vi "Reboot Active Target.vi"(8 "error in":errorcluster) -> (0 "error out":errorcluster)   [LabVIEW 2020, in "cRIO System Tests.lvclass"]
uses:
  cRIO System Tests.lvclass
  <vilib>/nisyscfg/nisyscfg.lvlib
  7f296576-305d-4d39-9592-3a047ecdf3ee.vi
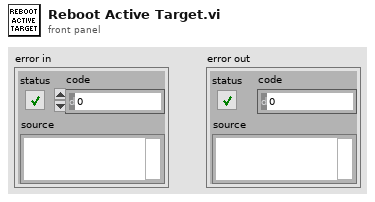
[diagram p1: front panel]
types:
  T1 = typedef "VeriStandTestUtilities.lvlib/TargetsConfiguration.ctl" = cluster{"Supported Targets":cluster{"IP Address / Hostname":string, "Target Platform":T2}[], "Active Configuration":T2}
  T2 = typedef "VeriStandTestUtilities.lvlib/TargetPlatform.ctl" = enum16{"Windows", "Linux64CRIO", "Linux64PXI", "LinuxARM", "PharLap"}
  T3 = cluster{"IP Address / Hostname":string, "Target Platform":T2}[]
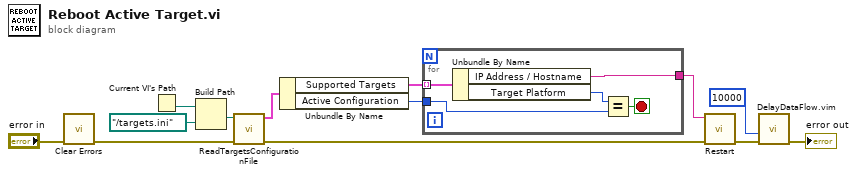
[diagram p0: block diagram]
diagram:
  n1 = call <vilib>:"Clear Errors.vi"("error in (no error)"="error in") -> ("error out"=w5:errorcluster)  [unwired: 5 in, 1 out]
  n2 = Current VI's Path() -> (path=w6:path)
  n3 = Build Path(base path=w6, name or relative path=path "../targets.ini") -> (appended path=w8:path)
  n4 = call <vilib>:"ReadTargetsConfigurationFile.vi"("error in (no error)"=w5, "targets.ini file"=w8) -> ("error out"=w13:errorcluster, "Targets Configuration"=w9:T1)  [unwired: 8 in]
  n5 = Unbundle By Name(w9) -> ("Supported Targets"=w10:T3, "Active Configuration"=w11:T2)
  n6 = for {
    tunnel: w10 -> [w18] mode=indexing
    tunnel: w11 -> [w16]
    tunnel: [w14] -> w12
    stop <- w15 stop-if-true
    n7 = Unbundle By Name(w18) -> ("IP Address / Hostname"=w14:string, "Target Platform"=w17:T2)
    n8 = Equal?(x=w17, y=w16) -> (x = y?=w15:bool)
  }
  n9 = call <vilib>:"Restart.vi"("error in (no error)"=w13, "Session in"=w12) -> ("error out"=w1:errorcluster)  [unwired: 7 in, 2 out]
  n10 = call "DelayDataFlow.vim"("value in"=w1, "milliseconds to wait"=u32 10000) -> ("value out"=→"error out":errorcluster)  [unwired: 2 in, 1 out]
